vi "RAW E2 Data.vi"() -> (0 "Read Data":T1)   [LabVIEW 2010, in "lib1299.lvlib"]
uses:
  lib1299.lvlib
  Controls/Read RAW data.ctl
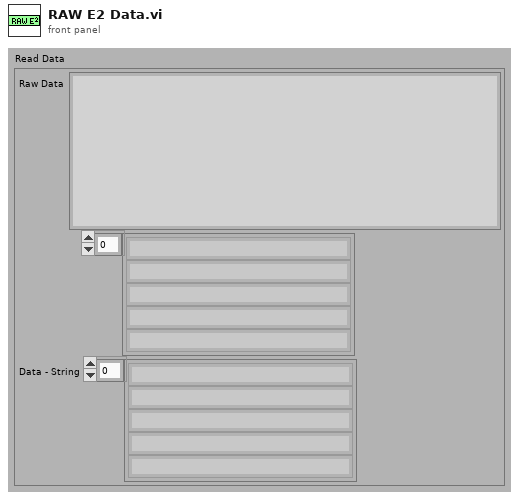
[diagram p1: front panel]
types:
  T1 = typedef "lib1299.lvlib/Read RAW data.ctl" = cluster{"Raw Data":string, "Parsed Data":string[], "Data - String":string[]}
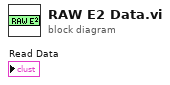
[diagram p0: block diagram]
diagram:
